vi "geve-populate_graph_data.vi"(8 "error in (no error)":errorcluster, 11 "Runtime Data":T1) -> (0 "error out":errorcluster, 3 "graph data":T5(array[cluster]))   [LabVIEW 2018]
doc: "populate graph data"
uses:
  geve-runtime_data_cluster.ctl
  geve-monitoring_data_cluster.ctl
  geve-serial_config_cluster.ctl
  geve-com_ref_cluster.ctl
  geve-message_cluster.ctl
  9c8ce9d9-92b9-4769-9d2a-39ea63119985.vi
  92c1334c-8e13-43bf-83e2-e54d05c77b77.vi
  bda35b2f-b66d-4909-8938-cf5606509624.vi
  87aab2d4-2adf-40f3-b6e4-0355fb32d9ce.vi
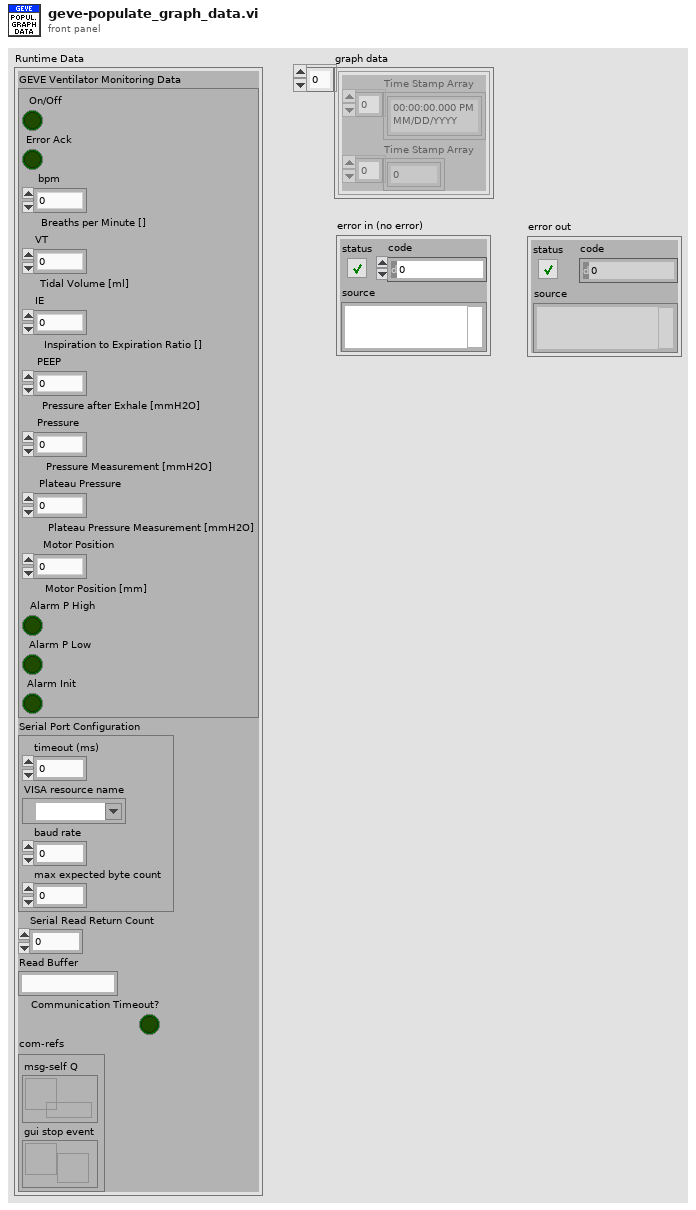
[diagram p1: front panel]
types:
  T1 = typedef "geve-runtime_data_cluster.ctl" = cluster{"GEVE Ventilator Monitoring Data":T2, "Serial Port Configuration":T3, "Serial Read Return Count":u32, "Read Buffer":string, "Communication Timeout?":bool, "com-refs":T4}
  T2 = typedef "geve-monitoring_data_cluster.ctl" = cluster{"On/Off":bool, "Error Ack":bool, "bpm":dbl, "VT":dbl, "IE":dbl, "PEEP":dbl, "Pressure":dbl, "Plateau Pressure":dbl, "Motor Position":dbl, "Alarm P High":bool, "Alarm P Low":bool, "Alarm Init":bool}
  T3 = typedef "geve-serial_config_cluster.ctl" = cluster{"timeout (ms)":u32, "VISA resource name":refnum<visa-resource-name>, "baud rate":u32, "max expected byte count":u32}
  T4 = typedef "geve-com_ref_cluster.ctl" = cluster{"msg-self Q":refnum<queue>, "gui stop event":refnum<user-event>}
  T5 = cluster{"Time Stamp Array":timestamp[], "Time Stamp Array":dbl[]}[]
  T6 = cluster{"Time Stamp Array":timestamp[], "Time Stamp Array":dbl[]}
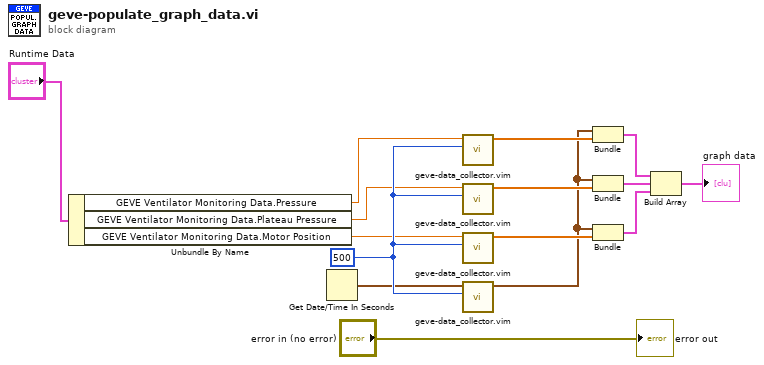
[diagram p0: block diagram]
diagram:
  w7 = 500 ("y")
  n1 = Unbundle By Name("Runtime Data") -> ("GEVE Ventilator Monitoring Data.Pressure"=w4:dbl, "GEVE Ventilator Monitoring Data.Plateau Pressure"=w5:dbl, "GEVE Ventilator Monitoring Data.Motor Position"=w6:dbl)
  n2 = Get Date/Time In Seconds() -> (seconds since 1Jan1904=w2:timestamp)
  n3 = call "geve-data_collector.vim"("Max Values"=w7, "Time Stamp"=w4) -> ("Time Stamp Array"=w13:dbl[])  [unwired: 9 in]
  n4 = call "geve-data_collector.vim"("Max Values"=w7, "Time Stamp"=w5) -> ("Time Stamp Array"=w14:dbl[])  [unwired: 9 in]
  n5 = call "geve-data_collector.vim"("Max Values"=w7, "Time Stamp"=w6) -> ("Time Stamp Array"=w15:dbl[])  [unwired: 9 in]
  n6 = call "geve-data_collector.vim"("Max Values"=w7, "Time Stamp"=w2) -> ("Time Stamp Array"=w12:timestamp[])  [unwired: 9 in]
  n7 = Bundle("Time Stamp Array"=w12, "Time Stamp Array"=w13) -> (w11:T6)  [unwired: 1 in]
  n8 = Bundle("Time Stamp Array"=w12, "Time Stamp Array"=w14) -> (w10:T6)  [unwired: 1 in]
  n9 = Bundle("Time Stamp Array"=w12, "Time Stamp Array"=w15) -> (w9:T6)  [unwired: 1 in]
  n10 = Build Array(w11, w10, w9) -> (→"graph data":T5)
  "error out" <- "error in (no error)"
